vi "from_bytes.vi"(11 "Bytes":refnum<class "Bytes.lvclass">) -> (3 "TypeDescriptor":refnum<class "TD.lvclass">)   [LabVIEW 2020, in "variant.lvlib" / "type.lvlib" / "TD.lvclass"]
uses:
  TD.lvclass
  Bytes/Bytes.lvclass
  Bytes/Bytes.lvclass/Bytes.ctl
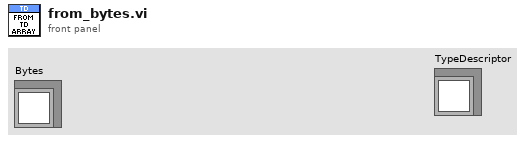
[diagram p1: front panel]
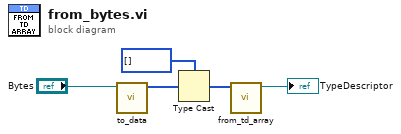
[diagram p0: block diagram]
diagram:
  n1 = call "to_data.vi"("Bytes in"="Bytes") -> ("byte array"=w5:u8[])  [unwired: 10 in]
  n2 = Type Cast(type=i16[] [] ("type descriptor array"), x=w5) -> (*(type *) &x=w4:i16[])
  n3 = call "from_td_array.vi"("type descriptor array"=w4) -> ("TypeDescriptor out"=→"TypeDescriptor":refnum<class "TD.lvclass">)  [unwired: 9 in, 1 out]
